vi "power out BAE7.vi"(0 "Max Voltage in (V)":dbl=8.5 format="%.2f", 7 "Normalized Power (0-1)":dbl format="%.2f", 11 "error in (no error)":errorcluster) -> (4 "Max Voltage out (V)":dbl=8.5 format="%.2f", 15 "error out":errorcluster)   [LabVIEW 2014]
doc: "power out BAE7\n\nCalculates the set voltage based off the max voltage and Normalized Power.\n\nVset = Vmax / ( Normalized Power)^(1/2) \n\nBeverly Abadines\nPHY 350\nE7"
panel:
  in  "Clear":bool
  in  "Device":tag="Dev1"
  # "Power Out BAE7"
  # "Beverly Abadines\nPhys 350\nE7"
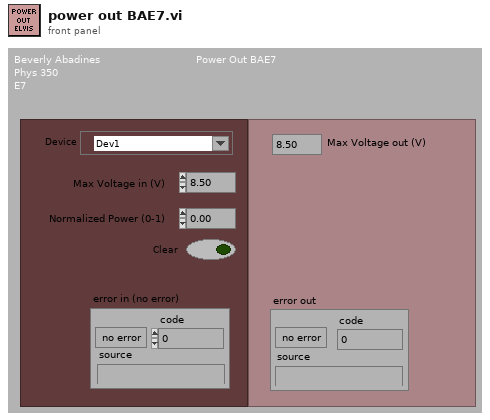
[diagram p1: front panel]
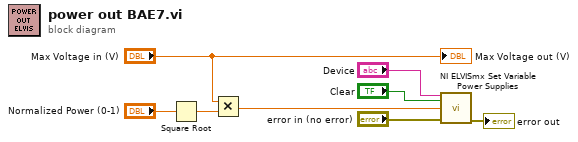
[diagram p0: block diagram]
diagram:
  n1 = Square Root(x="Normalized Power (0-1)") -> (sqrt(x)=w1:dbl)
  n2 = Multiply(x="Max Voltage in (V)", y=w1) -> (x*y=w2:dbl)
  n3 = call "NI ELVISmx Set Variable Power Supplies.vi"("Device Name"="Device", "Stop"="Clear", "Supply+ (V)"=w2, "error in"="error in (no error)") -> ("error out"=→"error out":errorcluster)  [unwired: 3 in, 12 out]
  "Max Voltage out (V)" <- "Max Voltage in (V)"
